vi "Create Project Item - Shared.vi"(8 "Error In":errorcluster, 11 "ProjectItem Refnum":refnum<vi>) -> (0 "Error Out":errorcluster, 1 "project_item":T1, 2 "Owned Items[]":refnum<vi>[](array[refnum]), 3 "ProjectItem Refnum Out":refnum<vi>)   [LabVIEW 2014, in "i3-docs.lvlib"]
uses:
  i3-docs.lvlib
  Controls/project_item.ctl
  Controls/image_information.ctl
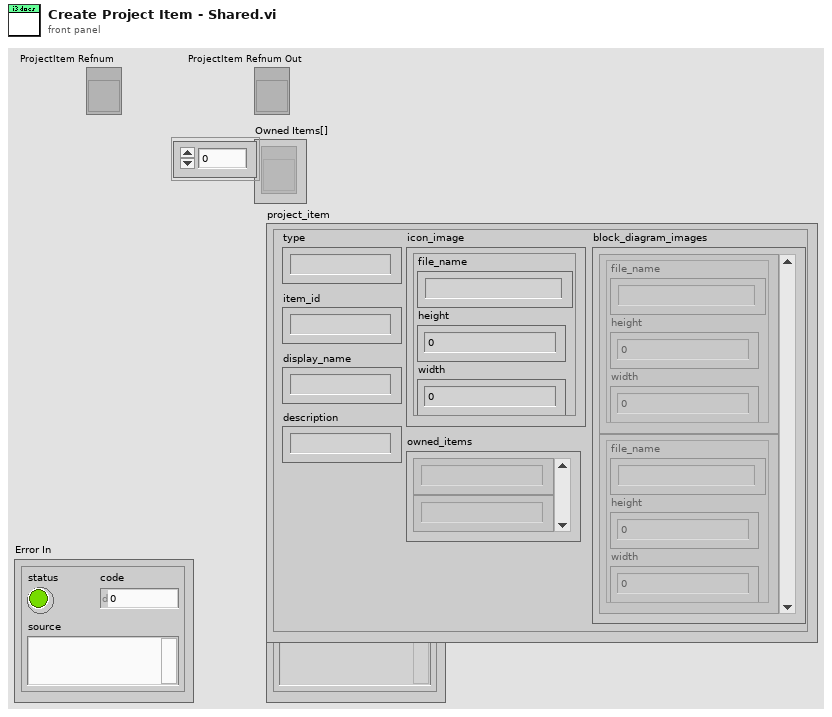
[diagram p1: front panel]
types:
  T1 = typedef "i3-docs.lvlib/project_item.ctl" = cluster{"type":string, "owned_items":string[], "item_id":string, "display_name":string, "description":string, "block_diagram_images":T2[], "icon_image":T2}
  T2 = typedef "i3-docs.lvlib/image_information.ctl" = cluster{"file_name":string, "height":i32, "width":i32}
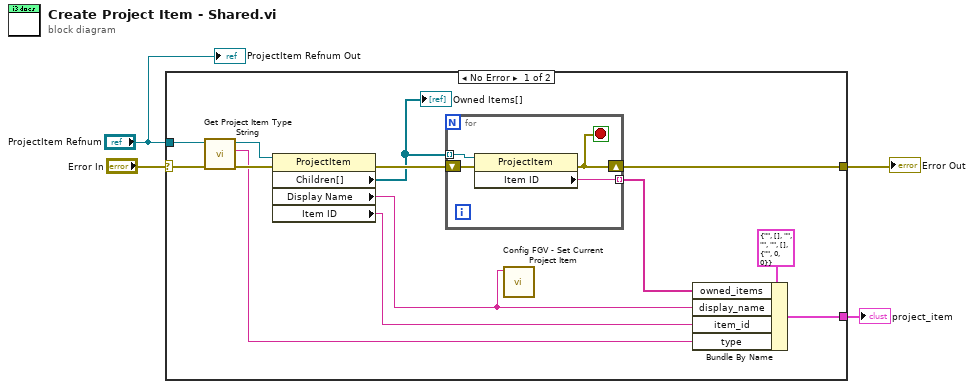
[diagram p0: block diagram]
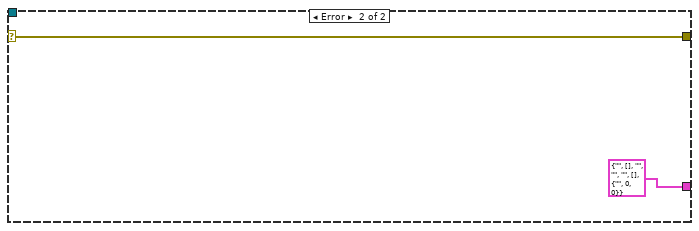
[diagram p2: hidden frame]
diagram:
  n1 = case shown="No Error" "Error In" {
    selector: "Error In" -> [w9 w23]
    tunnel: [w12 w23] -> w3
    tunnel: [w11 T1 {"type"="", "owned_items"=[], "item_id"="", "display_name"="", "description"="", "block_diagram_images"=[], "icon_image"={"file_name"="", "height"=0, "width"=0}} ("project_item")] -> w2
    tunnel: "ProjectItem Refnum" -> [w8 _]
    frame No Error {
      n2 = call "Get Project Item Type String.vi"("Error In"=w9, "ProjectItem Refnum"=w8) -> ("Error Out"=w10:errorcluster, "Type String"=w6:string, "ProjectItem Refnum Out"=w7:refnum<vi>)  [unwired: 7 in]
      n3 = property class="ProjectItem"(reference=w7, error in=w10) -> (error out=w17:errorcluster, "Children[]"=w16:refnum<vi>[], "Display Name"=w5:string, "Item ID"=w13:string)  [unwired: 1 out]
      "Owned Items[]" <- w16
      n4 = for {
        tunnel: w16 -> [w21] mode=indexing
        shift-right: [w19] -> w12
        shift-left: w17 -> [w20]
        tunnel: [w18] -> w14 mode=indexing
        stop <- w19 stop-if-true
        n5 = property class="ProjectItem"(reference=w21, error in=w20) -> (error out=w19:errorcluster, "Item ID"=w18:string)  [unwired: 1 out]
      }
      n6 = call "Config FGV - Set Current Project Item.vi"("Set Current Project Item"=w5) -> ()  [unwired: 11 in]
      n7 = Bundle By Name(cluster=T1 {"type"="", "owned_items"=[], "item_id"="", "display_name"="", "description"="", "block_diagram_images"=[], "icon_image"={"file_name"="", "height"=0, "width"=0}} ("project_item"), "owned_items"=w14, "display_name"=w5, "item_id"=w13, "type"=w6) -> (w11:T1)
    }
    frame Error {
    }
  }
  "Error Out" <- w3
  "project_item" <- w2
  "ProjectItem Refnum Out" <- "ProjectItem Refnum"
